vi "KE26XXA Advanced Sweep.vi"(0 "VISA resource name":refnum<visa-resource-name>, 1 "Channel":T1, 4 "Pulse Mode":bool, 5 "error in":errorcluster, 6 "Bias Level":dbl, 7 "Pulse Period":dbl=0.02, 8 "Start Value":dbl=1.0, 9 "Pulse Width":dbl=0.01, 10 "End Value":dbl=5.0, 11 "Points":u32=10 min=1, 12 "Limit":dbl=0.1) -> (16 "Data Out":dbl[](array[numeric]) format="%^#_6e", 19 "error out":errorcluster)   [LabVIEW 2012]
doc: "This example shows how to configure the advanced trigger model to perform a linear voltage sweep.\n\nThis example demonstrates the following:\n• Configuring sweeps\n• Configuring timers\n• Configuring SMU event modules\n• Linking event modules"
uses:
  Keithley 2600 Series.lvlib
  Instance           2 30Saved   KE26XXA Advanced Sweep .vi
  Instance           1 30Saved   KE26XXA Advanced Sweep .vi
  Public/Channel.ctl
panel:
  in  "Output Data":bool
  in  "Measurement":enum8{"DISABLE", "ENABLE", "ASYNC"}(ring)
  # "(c) 2008 Keithley Instruments, Inc.  ALL RIGHTS RESERVED."
  # "V"
  # "V"
  # "V"
  # "A"
  # "s"
  # "s"
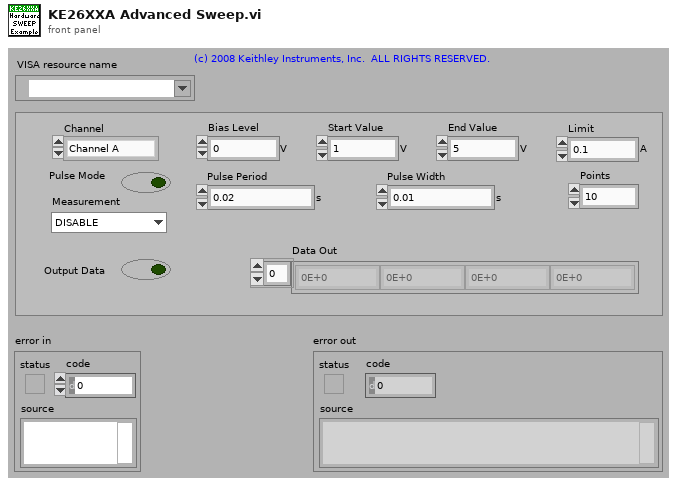
[diagram p1: front panel]
types:
  T1 = typedef "Keithley 2600 Series.lvlib/Channel.ctl" = enum32{"Channel A", "Channel B"}
  T2 = enum16{"Current", "Voltage", "IV", "Resistance", "Power"}
  T3 = enum16{"None/Disconnect", "Digital I/O Trigger", "TSP-Link Trigger", "LAN Trigger", "Blender", "Timer Expired", "Front Panel Trigger", "Software Trigger", "SMU Sweeping", "SMU Armed", "SMU Source Complete", "SMU Measure Complete", "SMU Pulse Complete", "SMU Sweep Complete", "SMU Idle"}
  T4 = enum32{"Digital I/O", "TSP-Link", "LAN", "Software"}
  T5 = enum16{"Linear Current", "Linear Voltage", "Logarithimic Current", "Logarithimic Voltage", "List Current", "List Voltage"}
  T6 = enum32{"Normal", "Big Endian", "Little Endian", "Network", "Swapped"}
  T7 = enum32{"ASCII", "Real 32", "Real 64", "Single Precision Real", "Double Precision Real"}
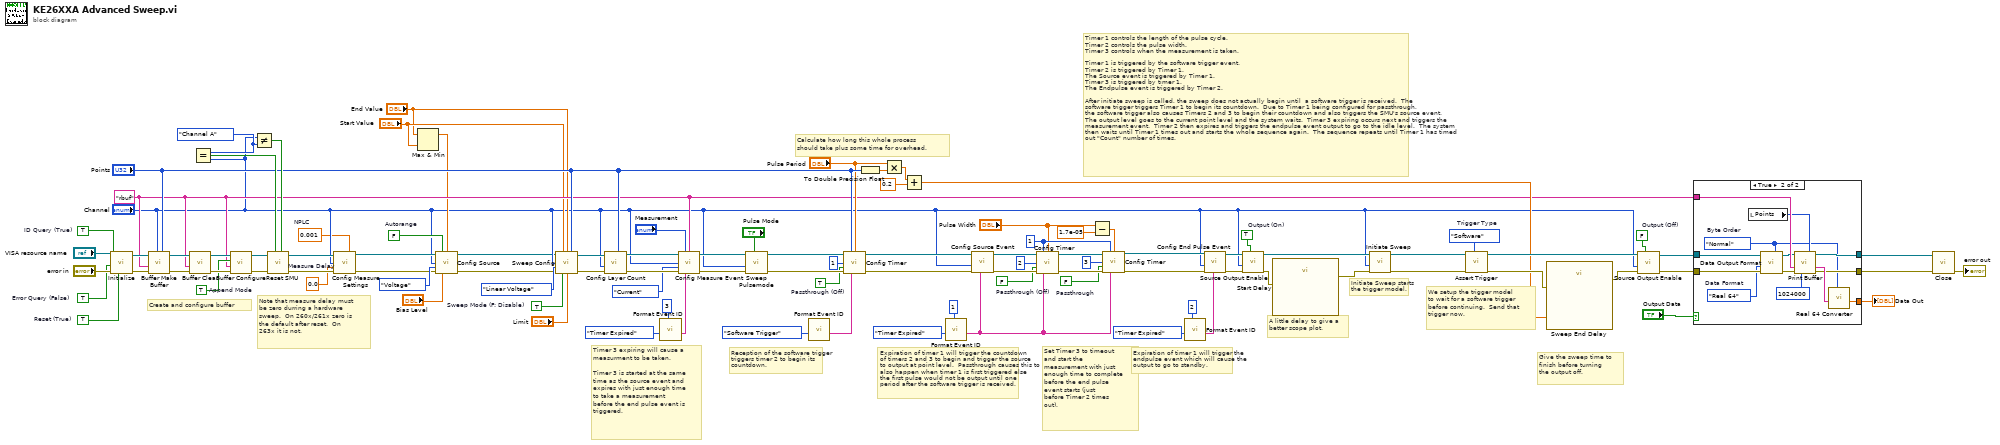
[diagram p0: block diagram]
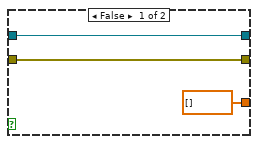
[diagram p2: hidden frame]
diagram:
  w7 = 0.0  # Measure Delay
  w5 = 0.001  # NPLC
  w20 = "rbuf"
  w23 = TRUE  # Append Mode
  w25 = Channel."Channel A" ("x")
  w38 = FALSE  # Passthrough
  w67 = FALSE  # Autorange
  w72 = TRUE  # Sweep Mode (F: Disable)
  w70 = TRUE  # Passthrough (Off)
  w68 = FALSE  # Passthrough (Off)
  w81 = FALSE  # Output (Off)
  w84 = TRUE  # Output (On)
  w87 = T4."Software"  # Trigger Type
  w90 = TRUE  # Reset (True)
  w91 = TRUE  # Error Query (False)
  w92 = TRUE  # ID Query (True)
  w42 = u32 1 ("Count")
  # "Note that measure delay must\nbe zero durring a hardware\nsweep.  On 260x/261x zero is\nthe default after reset.  On\n263x it is not."
  # "Set Timer 3 to timeout\nand start the\nmeasurement with just\nenough time to complete\nbefore the end pulse\nevent starts (just\nbefore Timer 2 times\nout)."
  # "Create and configure buffer"
  # "Calculate how long this whole process\nshould take plus some time for overhead."
  # "Timer 3 expiring will cause a\nmeasurment to be taken.\n\nTimer 3 is started at the same\ntime as the source event and\nexpires with just enough time\nto take a measurement\nbefore the end pulse event is\ntriggered."
  # "Give the sweep time to\nfinish before turning\nthe output off."
  # "A little delay to give a\nbetter scope plot."
  # "We setup the trigger model\nto wait for a software trigger\nbefore continuing.  Send that\ntrigger now."
  # "Reception of the software trigger\ntriggers timer 2 to begin its\ncountdown."
  # "Expiration of timer 1 will trigger the countdown\nof timers 2 and 3 to begin and trigger the source\nto output at point level.  Passthrough causes this to\nalso happen when timer 1 is first triggered else\nthe first pulse would not be output until one\nperiod after the software trigger is received."
  # "Expiration of timer 1 will trigger the\nendpulse event which will cause the\noutput to go to standby."
  # "Initiate Sweep starts\nthe trigger model."
  # "Timer 1 controls the length of the pulse cycle.\nTimer 2 controls the pulse width.\nTimer 3 controls when the measurement is taken.\n\nTimer 1 is triggered by the software trigger event.\nTimer 2 is triggered by Timer 1.\nThe Source event is triggered by Timer 1.\nTimer 3 is triggered by timer 1.\nThe Endpulse event is triggered by Timer 2.\n\nAfter initiate sweep is called, the sweep does not actually begin until  a software trigger is received.  The\nsoftware trigger triggers Timer 1 to begin its countdown.  Due to Timer 1 being configured for passthrough,\nthe software trigger also causes Timers 2 and 3 to begin their countdown and also triggers the SMU's source event.\nThe output level goes to the current point level and the system waits.  Timer 3 expiring occurs next and triggers the\nmeasurement event.  Timer 2 then expires and triggers the endpulse event output to go to the idle level.  The system\nthen waits until Timer 1 times out and starts the whole sequence again.  The sequence repeats until Timer 1 has timed\nout \"Count\" number of times."
  n1 = call "Initialize.vi"("Reset (True)"=w90, "error in (no error)"="error in", "Error Query (False)"=w91, "ID Query (True)"=w92, "VISA resource name"="VISA resource name") -> ("error out"=w35:errorcluster, "VISA resource name out"=w28:refnum<visa-resource-name>)  [unwired: 1 in, 4 out]
  n2 = call "Buffer Make Buffer.vi"("Capacity (1)"="Points", "Channel (Channel A)"="Channel", "error in (no error)"=w35, "Buffer Name (buf)"=w20, "VISA resource name"=w28) -> ("error out"=w34:errorcluster, "VISA resource name out"=w29:refnum<visa-resource-name>)  [unwired: 1 in, 4 out]
  n3 = call "Buffer Clear.vi"("error in (no error)"=w34, "Buffer Name"=w20, "VISA resource name"=w29) -> ("error out"=w33:errorcluster, "VISA resource name out"=w30:refnum<visa-resource-name>)  [unwired: 7 out]
  n4 = Equal?(x=w25, y="Channel") -> (x = y?=w27:bool)
  n5 = call "Buffer Configure.vi"("error in (no error)"=w33, "Buffer Name"=w20, "Append Mode (Off)"=w23, "VISA resource name"=w30) -> ("error out"=w32:errorcluster, "VISA resource name out"=w31:refnum<visa-resource-name>)  [unwired: 3 in, 3 out]
  n6 = Not Equal?(x="Channel", y=w25) -> (x != y?=w26:bool)
  n7 = call "Reset SMU.vi"("SMU B (No)"=w26, "SMU A (No)"=w27, "error in (no error)"=w32, "VISA resource name"=w31) -> ("error out"=w10:errorcluster, "VISA resource name out"=w11:refnum<visa-resource-name>)  [unwired: 1 in, 5 out]
  n8 = call "Config Measure Settings.vi"("VISA resource name"=w11, "NPLC (1.000)"=w5, "Channel (Channel A)"="Channel", "Measure Delay (0)"=w7, "error in"=w10) -> ("VISA resource name out"=w9:refnum<visa-resource-name>, "error out"=w8:errorcluster)  [unwired: 5 in, 4 out]
  n9 = Max & Min(x="End Value", y="Start Value") -> (max(x,y)=w12:dbl)  [unwired: 1 out]
  n10 = call "Config Source.vi"("VISA resource name"=w9, "Autorange (On)"=w67, "Range (1.000)"=w12, "Channel (Channel A)"="Channel", "Function (Current)"=enum32{"Current", "Voltage"}."Voltage", "error in"=w8, "Level (0.000)"="Bias Level") -> ("VISA resource name out"=w4:refnum<visa-resource-name>, "error out"=w3:errorcluster)  [unwired: 4 in, 3 out]
  n11 = call "Sweep Config.vi"("VISA resource name"=w4, "Start Value"="Start Value", "End Value"="End Value", "Points (1)"="Points", "Channel (Channel A)"="Channel", "Sweep Type"=T5."Linear Voltage", "error in"=w3, "Sweep Mode (F: Disable)"=w72, "Limit (0.1)"="Limit") -> ("VISA resource name out"=w80:refnum<visa-resource-name>, "error out"=w79:errorcluster)  [unwired: 2 in, 3 out]
  n12 = call "Config Layer Count.vi"("Trigger Count (1)"="Points", "error in"=w79, "Channel (Channel A)"="Channel", "VISA resource name"=w80) -> ("error out"=w58:errorcluster, "VISA resource name out"=w57:refnum<visa-resource-name>)  [unwired: 2 in, 4 out]
  n13 = call "Format Event ID.vi"("Event Module # (1)"=u32 3, "Event Type (None)"=T3."Timer Expired") -> ("Event ID"=w53:string)  [unwired: 2 in, 7 out]
  n14 = call "Config Measure Event.vi"("VISA resource name"=w57, "Configure Measurement (Disable)"="Measurement", "Buffer 1"=w20, "Channel (Channel A)"="Channel", "Function (Current)"=T2."Current", "error in"=w58, "Measure Input Event"=w53) -> ("VISA resource name out"=w56:refnum<visa-resource-name>, "error out"=w55:errorcluster)  [unwired: 2 in, 5 out]
  n15 = call "Sweep Pulsemode.vi"("Pulse Mode (F: Disabled)"="Pulse Mode", "error in"=w55, "Channel (Channel A)"="Channel", "VISA resource name"=w56) -> ("error out"=w74:errorcluster, "VISA resource name out"=w73:refnum<visa-resource-name>)  [unwired: 1 in, 5 out]
  n16 = call "Format Event ID.vi"("Event Type (None)"=T3."Software Trigger") -> ("Event ID"=w69:string)  [unwired: 3 in, 7 out]
  n17 = call "Config Timer.vi"("VISA resource name"=w73, "Count (1)"="Points", "Delay (1e-3)"="Pulse Period", "Timer Number (1)"=u32 1, "Passthrough (Off)"=w70, "error in"=w74, "Input Event"=w69) -> ("VISA resource name out"=w45:refnum<visa-resource-name>, "error out"=w46:errorcluster)  [unwired: 2 in, 5 out]
  n18 = To Double Precision Float(number="Points") -> (double precision float=w22:dbl)
  n19 = Multiply(x="Pulse Period", y=w22) -> (x*y=w36:dbl)
  n20 = Add(x=w36, y=0.2 ("x")) -> (x+y=w60:dbl)
  n21 = call "Format Event ID.vi"("Event Module # (1)"=u32 1, "Event Type (None)"=T3."Timer Expired") -> ("Event ID"=w43:string)  [unwired: 2 in, 7 out]
  n22 = call "Config Timer.vi"("VISA resource name"=w45, "Count (1)"=w42, "Delay (1e-3)"="Pulse Width", "Timer Number (1)"=u32 2, "Passthrough (Off)"=w68, "error in"=w46, "Input Event"=w43) -> ("VISA resource name out"=w75:refnum<visa-resource-name>, "error out"=w76:errorcluster)  [unwired: 2 in, 5 out]
  n23 = call "Config Source Event.vi"("Input Event"=w43, "error in"=w76, "Channel (Channel A)"="Channel", "VISA resource name"=w75) -> ("error out"=w50:errorcluster, "VISA resource name out"=w49:refnum<visa-resource-name>)  [unwired: 1 in, 5 out]
  n24 = Subtract(x="Pulse Width", y=1.7e-05) -> (x-y=w40:dbl)
  n25 = call "Config Timer.vi"("VISA resource name"=w49, "Count (1)"=w42, "Delay (1e-3)"=w40, "Timer Number (1)"=u32 3, "Passthrough (Off)"=w38, "error in"=w50, "Input Event"=w43) -> ("VISA resource name out"=w48:refnum<visa-resource-name>, "error out"=w47:errorcluster)  [unwired: 2 in, 5 out]
  n26 = call "Format Event ID.vi"("Event Module # (1)"=u32 2, "Event Type (None)"=T3."Timer Expired") -> ("Event ID"=w98:string)  [unwired: 2 in, 7 out]
  n27 = call "Config End Pulse Event.vi"("Input Event"=w98, "error in"=w47, "Channel (Channel A)"="Channel", "VISA resource name"=w48) -> ("error out"=w85:errorcluster, "VISA resource name out"=w86:refnum<visa-resource-name>)  [unwired: 1 in, 5 out]
  n28 = call "Source Output Enable.vi"("Output (Off)"=w84, "error in (no error)"=w85, "Channel (Channel A)"="Channel", "VISA resource name"=w86) -> ("error out"=w64:errorcluster, "VISA resource name out"=w83:refnum<visa-resource-name>)  [unwired: 1 in, 5 out]
  n29 = call "Start Delay"("error in (no error)"=w64) -> ("error out"=w63:errorcluster)  [unwired: 1 in, 9 out]
  n30 = call "Initiate Sweep.vi"("error in"=w63, "Channel (Channel A)"="Channel", "VISA resource name"=w83) -> ("error out"=w89:errorcluster, "VISA resource name out"=w88:refnum<visa-resource-name>)  [unwired: 1 in, 6 out]
  n31 = call "Assert Trigger.vi"("Trigger Type (Digital I/O)"=w87, "error in"=w89, "VISA resource name"=w88) -> ("error out"=w61:errorcluster, "VISA resource name out"=w82:refnum<visa-resource-name>)  [unwired: 2 in, 5 out]
  n32 = call "Sweep End Delay"("error in (no error)"=w61, "Delay Time (s)"=w60) -> ("error out"=w62:errorcluster)  [unwired: 9 out]
  n33 = call "Source Output Enable.vi"("Output (Off)"=w81, "error in (no error)"=w62, "Channel (Channel A)"="Channel", "VISA resource name"=w82) -> ("error out"=w19:errorcluster, "VISA resource name out"=w18:refnum<visa-resource-name>)  [unwired: 1 in, 5 out]
  n34 = case shown="True" "Output Data" {
    tunnel: w20 -> [_ w118]
    tunnel: w19 -> [w104 w117]
    tunnel: w18 -> [w105 w116]
    tunnel: [dbl[] [] ("Data Array Out") w112] -> w17
    tunnel: [w105 w109] -> w16
    tunnel: [w104 w108] -> w15
    frame False {
    }
    frame True {
      w107 = T6."Normal"  # Byte Order
      w110 = T7."Real 64"  # Data Format
      n35 = local read "Points"() -> (w111:u32)
      n36 = call "Data Output Format.vi"("Byte Order (Normal)"=w107, "error in (no error)"=w117, "Data Format (ASCII)"=w110, "VISA resource name"=w116) -> ("error out"=w114:errorcluster, "VISA resource name out"=w115:refnum<visa-resource-name>)  [unwired: 2 in, 4 out]
      n37 = call "Print Buffer.vi"("VISA resource name"=w115, "End Index (1)"=w111, "Buffer Name(s)"=w118, "error in (no error)"=w114, "Byte Count (1024)"=u32 1024000) -> ("VISA resource name out"=w109:refnum<visa-resource-name>, "Buffer Data"=w113:string, "error out"=w108:errorcluster)  [unwired: 2 in, 6 out]
      n38 = call "Real 64 Converter.vi"("Byte Order (Normal)"=w107, "Data In"=w113) -> ("Data Array Out"=w112:dbl[])  [unwired: 9 out]
    }
  }
  "Data Out" <- w17
  n39 = call "Close.vi"("error in (no error)"=w15, "VISA resource name"=w16) -> ("error out"=→"error out":errorcluster)  [unwired: 9 out]
